vi "WaitRT_us.vi"(7 "Time to wait":i32 caption="Time to wait [µs]" min=0, 9 "Skip wait on error?":bool=TRUE caption="Skip wait on error? (T)", 11 "Error in":errorcluster caption="Error in (no error)", 12 "Skip wait?":bool caption="Skip wait? (F)") -> (15 "Error out":errorcluster)   [LabVIEW 2017, in "GPTiming.lvlib"]
doc: "Waits <B>Time to wait</B>. Select a polymorphic instance of either hours, minutes, seconds, milliseconds, milliseconds (Real-Time) or microseconds (Real-Time) by right-clicking the function.\n\n<B>Time to wait</B> is an I32 to have better type compatibility with other integer calculations in LabVIEW. If <B>Time to wait</B> is negative, it will be coerced to zero.\n\nThis VI is inlined. It skips the wait if there is an error on <B>Error in</B> and <B>Skip wait on error?</B> is True (which is the default). It also skips the wait unconditionally if <B>Skip wait?</B> is True.\n\n<B>Note</B>\nThe non-Real-Time version (which works both on Desktop and on Real-Time) of this function yields control of the execution thread during the wait, but it behaves differently on Windows and on Real-Time. On Windows, the function waits up to the value specified in <B>Time to wait</B>. On Real-Time the function waits at least the value specified in <B>Time to wait</B>. This function has a margin of error of plus or minus one millisecond.\n\n<B>Note</B> (Real-Time)\nThe Real-Time versions of this function blocks the execution of the thread of the calling VI. Any code running in parallel in the calling VI or any VIs running in the same execution system thread are unable to execute during the time that these functions wait.\n\nSteen Schmidt\nGPower\n1/1 2013"
uses:
  GPTiming.lvlib
  Error/GPError.lvlib
panel:
  # "Copyright © 2014\nGPower\nSee enclosed license file for terms and conditions"
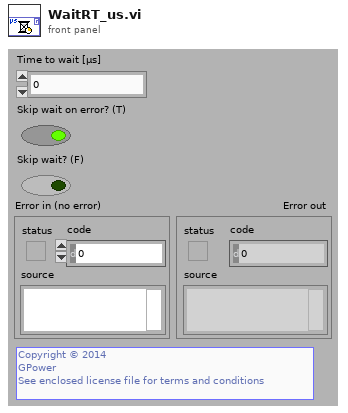
[diagram p1: front panel]
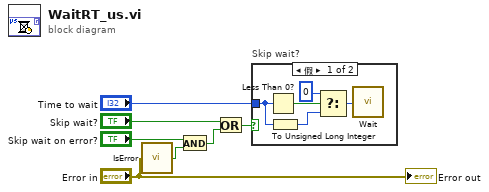
[diagram p0: block diagram]
diagram:
  n1 = call "IsError.vi"("Error in"="Error in") -> ("Error?"=w5:bool)  [unwired: 4 in]
  n2 = And(x="Skip wait on error?", y=w5) -> (x .and. y?=w3:bool)
  n3 = Or(x="Skip wait?", y=w3) -> (x .or. y?=w2:bool)
  n4 = case "Skip wait?" shown="假" w2 {
    tunnel: "Time to wait" -> [w12 _]
    frame False {
      n5 = Less Than 0?(x=w12) -> (x < 0?=w11:bool)
      n6 = To Unsigned Long Integer(number=w12) -> (unsigned 32bit integer=w10:u32)
      n7 = Select(t=u32 0, s=w11, f=w10) -> (s? t:f=w8:u32)
      n8 = call "Wait"("Count(uSec)"=w8) -> ()  [unwired: 1 out]
    }
    frame True {
    }
  }
  "Error out" <- "Error in"
